vi "Find Gasbottle CompIndex by similar CompName.vi"(10 "Botle Index":u32, 11 "Comp Name":string) -> (0 "Genauigkeit":dbl, 1 "Einheit":string, 2 "Konzentration IST":dbl, 3 "Gas Component Index in Bottle":i32, 4 "Komplette Übereinstimmung":string, 6 "Komplette Übereinstimmung Bottle":string, 7 "Komponenten":T1[](array[typedef]) {"Konzentration IST" format="%#.4f"; "Genauigkeit" format="%#.1f"})   [LabVIEW 2020, in "System Einstellungen V2.lvlib"]
uses:
  System Einstellungen V2.lvlib
  Gasflaschenkomponente.ctl
  Aktion FGV Gasbottledefinition.ctl
  <vilib>/regexp/Match Regular Expression.xnode
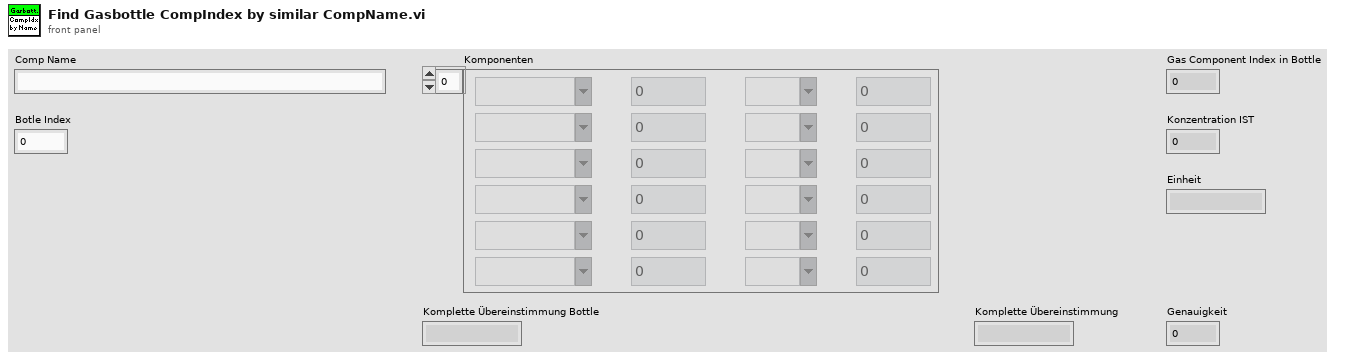
[diagram p1: front panel]
types:
  T1 = typedef "System Einstellungen V2.lvlib/Gasflaschenkomponente.ctl" = cluster{"Gasauswahl":string, "Konzentration IST":dbl, "Einheit":string, "Genauigkeit":dbl}
  T2 = typedef "System Einstellungen V2.lvlib/Aktion FGV Gasbottledefinition.ctl" = enum16{"lesen", "schreiben", "löschen", "laden", "speichern", "exportieren", "importieren"}
  T3 = typedef "System Einstellungen V2.lvlib/Gasflasche gesamt.ctl" = cluster{"Gasflasche":T4, "Trägergas":T5, "Komponenten":T1[]}
  T4 = typedef "System Einstellungen V2.lvlib/Gasflasche.ctl" = cluster{"Gasname für die Auswahl":string, "Chargennummer":string, "Ablaufdatum":timestamp}
  T5 = typedef "System Einstellungen V2.lvlib/Traegergas.ctl" = string
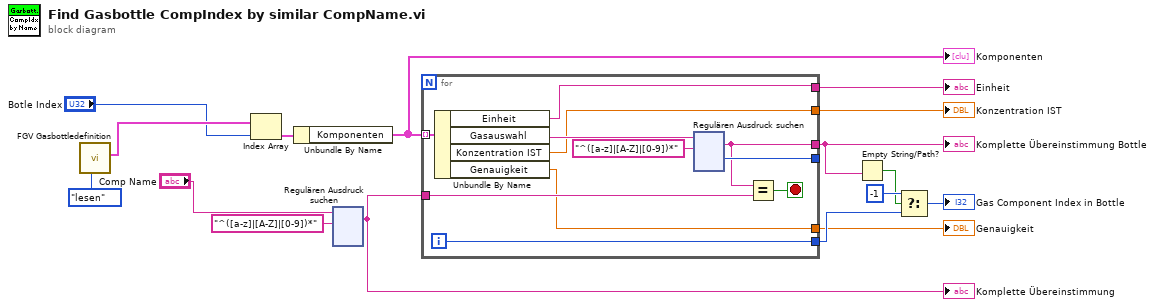
[diagram p0: block diagram]
diagram:
  n1 = call "FGV Gasbottledefinition.vi"("Aktion"=Aktion_FGV_Gasbottledefinition."lesen") -> ("Gasflaschen Liste gesamt"=w13:T3[])  [unwired: 8 in, 2 out]
  n2 = Index Array(array=w13, index="Botle Index") -> (element=w11:T3)
  n3 = Unbundle By Name(w11) -> ("Komponenten"=w10:T1[])
  "Komponenten" <- w10
  n4 = xnode "Regulären Ausdruck suchen"("Eingangs-String"="Comp Name", "Regulärer Ausdruck"="^([a-z]|[A-Z]|[0-9])*") -> ("Komplette Übereinstimmung"=w9:string)  [unwired: 4 in, 4 out]
  "Komplette Übereinstimmung" <- w9
  n5 = for {
    tunnel: w10 -> [w27] mode=indexing
    tunnel: w9 -> [w24]
    tunnel: [w22] -> w8
    tunnel: [w21] -> _
    tunnel: [w20] -> w5
    tunnel: [w19] -> w3
    tunnel: [w18] -> w2
    tunnel: [w17] -> w1
    i -> [w22]
    stop <- w23 stop-if-true
    n6 = Unbundle By Name(w27) -> ("Einheit"=w18:string, "Gasauswahl"=w25:string, "Konzentration IST"=w19:dbl, "Genauigkeit"=w17:dbl)
    n7 = xnode "Regulären Ausdruck suchen"("Eingangs-String"=w25, "Regulärer Ausdruck"="^([a-z]|[A-Z]|[0-9])*") -> ("Komplette Übereinstimmung"=w20:string, "Offset nach Übereinstimmung"=w21:i32)  [unwired: 4 in, 3 out]
    n8 = Equal?(x=w20, y=w24) -> (x = y?=w23:bool)
  }
  "Komplette Übereinstimmung Bottle" <- w5
  "Konzentration IST" <- w3
  "Einheit" <- w2
  "Genauigkeit" <- w1
  n9 = Empty String/Path?(string/path=w5) -> (empty?=w4:bool)
  n10 = Select(t=-1 ("f"), s=w4, f=w8) -> (s? t:f=→"Gas Component Index in Bottle":i32)
